vi "writeBoolean.vi"(8 "error in (no error)":errorcluster, 10 "Input":bool, 11 "M1M3SAL in":refnum<class "M1M3SAL.lvclass">) -> (0 "error out":errorcluster, 3 "M1M3SAL out":refnum<class "M1M3SAL.lvclass">)   [LabVIEW 2016, in "M1M3SupportCommunicator.lvlib" / "M1M3SAL.lvclass"]
uses:
  M1M3SAL.lvclass
  M1M3SAL.lvclass/M1M3SAL.ctl
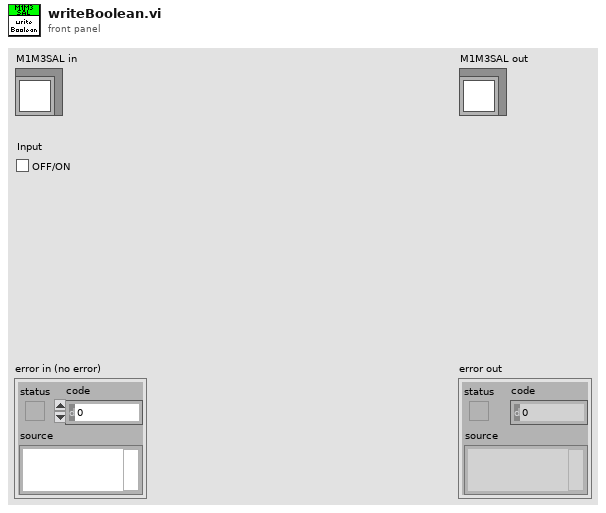
[diagram p1: front panel]
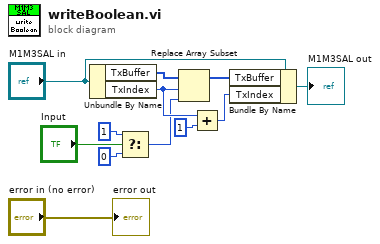
[diagram p0: block diagram]
diagram:
  n1 = Unbundle By Name("M1M3SAL in") -> ("TxBuffer"=w10:u8[], "TxIndex"=w9:i32)
  n2 = Select(t=u8 1 ("new element/subarray"), s="Input", f=u8 0 ("new element/subarray")) -> (s? t:f=w1:u8)
  n3 = Replace Array Subset(array=w10, new element=w1, index=w9) -> (w6:u8[])
  n4 = Add(x=w9, y=1) -> (x+y=w7:i32)
  n5 = Bundle By Name(cluster="M1M3SAL in", "TxBuffer"=w6, "TxIndex"=w7) -> (→"M1M3SAL out":refnum<class "M1M3SAL.lvclass">)
  "error out" <- "error in (no error)"
